vi "dfd_Lattice ARMA Normalization (Norm).vi"(7 "scale type":T1, 9 "coefficients v":dbl[](array[numeric]) format="%.2f", 10 "coefficients k":dbl[](array[numeric]) format="%.2f", 11 "x":dbl[](array[numeric])) -> (2 "norm":dbl[](array[numeric]) format="%.2f", 3 "y":dbl[](array[numeric]))   [LabVIEW 2017, in "NI_DigFilter_FXP.lvlib"]
uses:
  <vilib>/addons/Digital Filter Design/NI_DigFilter_FXP.lvlib
  <vilib>/addons/Digital Filter Design/_Objects.llb/DFD Coef Norm Type.ctl
  <vilib>/addons/Digital Filter Design/NI_DigFilterLicensed.lvlib
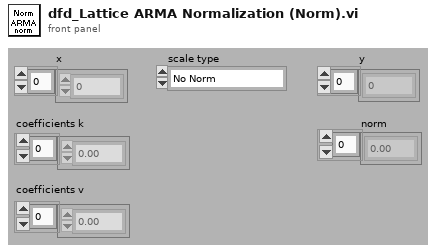
[diagram p1: front panel]
types:
  T1 = typedef "NI_DigFilterLicensed.lvlib/DFD Coef Norm Type.ctl" = enum16{"No Norm", "Time Domain 1-Norm", "Time Domain 2-Norm", "Time Domain Inf-Norm"}
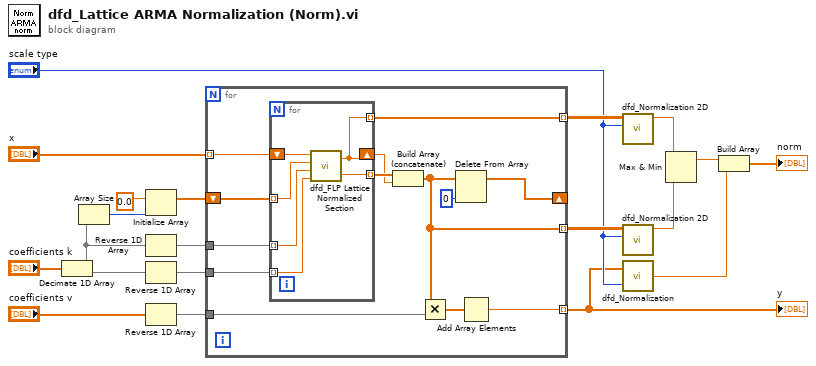
[diagram p0: block diagram]
diagram:
  n1 = Decimate 1D Array("coefficients k") -> (w4:dbl[], w2:dbl[])
  n2 = Array Size(array=w4) -> (size(s)=w19:i32)
  n3 = Initialize Array(0.0 ("element"), w19) -> (w20:dbl[])
  n4 = Reverse 1D Array(array=w4) -> (reversed array=w18:dbl[])
  n5 = Reverse 1D Array(array=w2) -> (reversed array=w1:dbl[])
  n6 = Reverse 1D Array(array="coefficients v") -> (reversed array=w17:dbl[])
  n7 = for {
    tunnel: w18 -> [w33]
    shift-right: [w28] -> _
    shift-left: w20 -> [w32]
    tunnel: [w22] -> w5 mode=indexing
    tunnel: w17 -> [w27]
    tunnel: [w26] -> w11 mode=indexing
    tunnel: [w25] -> w10 mode=indexing
    tunnel: "x" -> [w24] mode=indexing
    tunnel: w1 -> [w21]
    n8 = for {
      shift-right: [w38] -> w30
      shift-left: w24 -> [w39]
      tunnel: w32 -> [w36] mode=indexing
      tunnel: w33 -> [w35] mode=indexing
      tunnel: [w37] -> w31 mode=indexing
      tunnel: [w38] -> w26 mode=indexing
      tunnel: w21 -> [w34] mode=indexing
      n9 = call <vilib>:"dfd_FLP Lattice Normalized Section.vi"("^k(m)"=w34, "k(m)"=w35, "w(m-1)"=w36, "x(m)"=w39) -> ("w(m)"=w37:dbl, "x(m-1)"=w38:dbl)
    }
    n10 = Build Array (concatenate)(w31, w30) -> (w25:dbl[])
    n11 = Multiply(x=w25, y=w27) -> (x*y=w23:dbl[])
    n12 = Delete From Array(array=w25, index=0) -> (array with subset deleted=w28:dbl[])  [unwired: 1 in, 1 out]
    n13 = Add Array Elements(numeric array=w23) -> (sum=w22:dbl)
  }
  "y" <- w5
  n14 = call <vilib>:"dfd_Normalization 2D.vi"("scale type"="scale type", "2D Array (col-major)"=w11) -> ("max norm"=w9:dbl)  [unwired: 9 out]
  n15 = call <vilib>:"dfd_Normalization 2D.vi"("scale type"="scale type", "2D Array (col-major)"=w10) -> ("max norm"=w8:dbl)  [unwired: 9 out]
  n16 = call <vilib>:"dfd_Normalization.vi"("scale type"="scale type", "h(n)"=w5) -> ("norm"=w14:dbl)
  n17 = Max & Min(x=w9, y=w8) -> (max(x,y)=w6:dbl)  [unwired: 1 out]
  n18 = Build Array(w6, w14) -> (→"norm":dbl[])
